vi "CLAW_PID.vi"() -> ()   [LabVIEW 2013]
uses:
  <vilib>/addons/control/pid/pid.llb/PID (DBL).vi
  <vilib>/addons/control/pid/NI_PID_pid.lvlib
panel:
  out "In Range?":bool
  in  "Max_Analog_Volts":dbl=5.0 format="%#_13g"
  out "Waveform Chart":dbl(graph)
  in  "CLAW_Neutral_Position":dbl=2.5 format="%#_13g"
  in  "Analog_Input":dbl(slide) scale=0.0..5.0
  out "Motor_Output":dbl(knob) scale=-1.0..1.0
  in  "JoyStick":dbl(slide) scale=-1.0..1.0
  in  "Arm_Extend_Limit":dbl(slide)=4.36 scale=1.0..-1.0
  in  "Arm_Retract_Limit":dbl(slide)=0.6 scale=1.0..-1.0
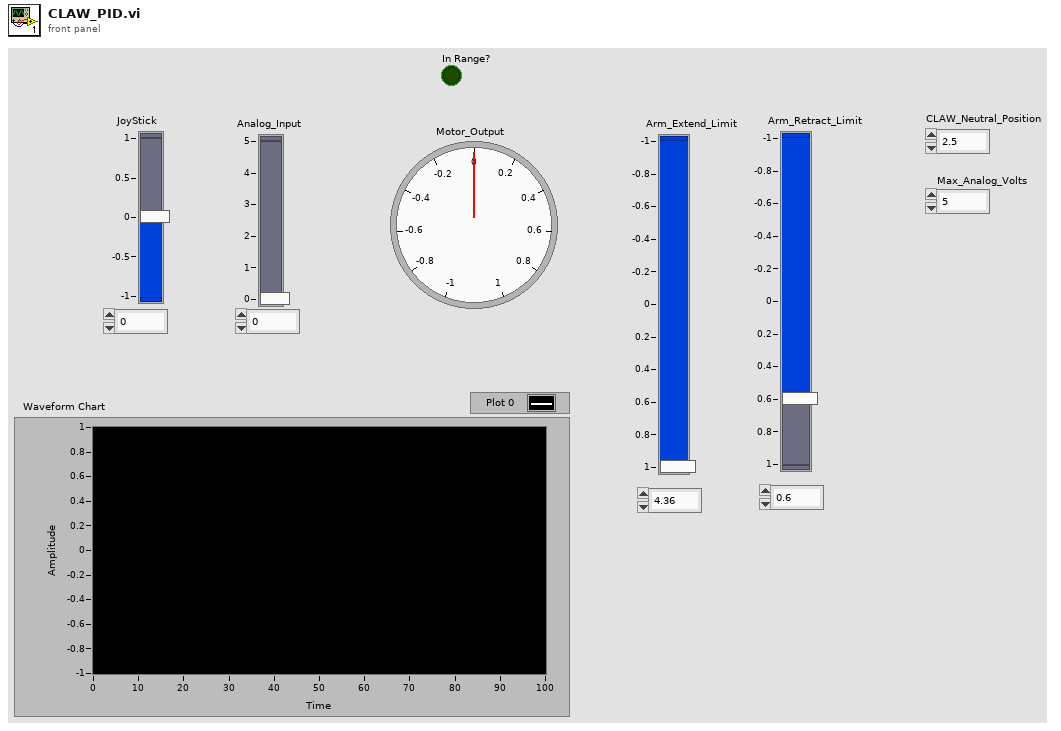
[diagram p1: front panel]
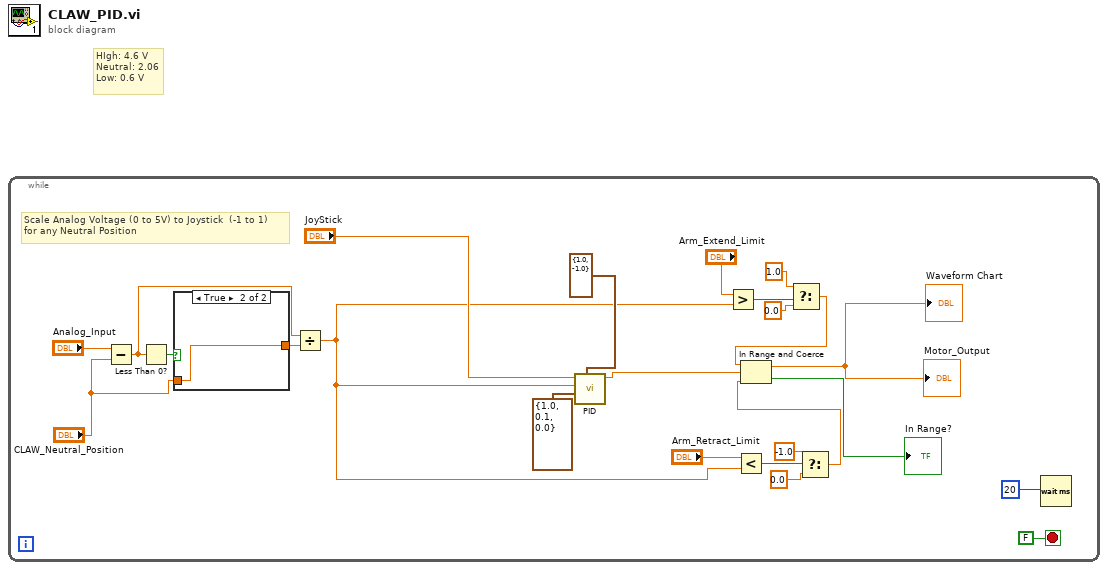
[diagram p0: block diagram]
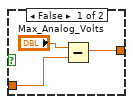
[diagram p2: hidden frame]
diagram:
  # "HIgh: 4.6 V\nNeutral: 2.06\nLow: 0.6 V"
  n1 = while {
    stop <- FALSE stop-if-true
    # "Scale Analog Voltage (0 to 5V) to Joystick  (-1 to 1)\nfor any Neutral Position"
    n2 = Subtract(x="Analog_Input", y="CLAW_Neutral_Position") -> (x-y=w15:dbl)
    n3 = Less Than 0?(x=w15) -> (x < 0?=w17:bool)
    n4 = case shown="True" w17 {
      tunnel: "CLAW_Neutral_Position" -> [w26 w28]
      tunnel: [w25 w28] -> w14
      frame False {
        n5 = Subtract(x="Max_Analog_Volts", y=w26) -> (x-y=w25:dbl)
      }
      frame True {
      }
    }
    n6 = Divide(x=w15, y=w14) -> (x/y=w18:dbl)
    n7 = call-poly <vilib>:"PID.vi"("output range"=cluster{"output low":dbl, "output high":dbl} {"output low"=1.0, "output high"=-1.0}, "PID gains"=cluster{dbl, dbl, dbl} {1.0, 0.1, 0.0}, "process variable"=w18, "setpoint"="JoyStick") -> ("output"=w5:dbl)  [unwired: 2 in, 5 out]
    n8 = Greater?(x="Arm_Extend_Limit", y=w18) -> (0:w12:bool)
    n9 = Less?(x="Arm_Retract_Limit", y=w18) -> (x < y?=w9:bool)
    n10 = Select(t=1.0, s=w12, f=0.0) -> (s? t:f=w2:dbl)
    n11 = Select(t=-1.0, s=w9, f=0.0) -> (s? t:f=w1:dbl)
    n12 = In Range and Coerce(upper limit=w2, x=w5, lower limit=w1) -> (coerced(x)=→"Motor_Output" →"Waveform Chart":dbl, In Range?=→"In Range?":bool)
    n13 = Wait (ms)(milliseconds to wait=20) -> ()  [unwired: 1 out]
  }
